vi "Launch Instruments.vi"(8 "error in (no error)":errorcluster, 11 "gController in":refnum<class "gController.lvclass">) -> (0 "error out":errorcluster, 3 "gController out":refnum<class "gController.lvclass">)   [LabVIEW 2017, in "Controller.lvlib" / "gController.lvclass"]
uses:
  gController.lvclass
  C:/Program Files (x86)/National Instruments/LabVIEW 2017/vi.lib/MSR Consulting, LLC/General Reuse/SuperActor/SuperActor.lvclass
  PAS/nPAS.lvclass
  C:/Program Files (x86)/National Instruments/LabVIEW 2017/vi.lib/MSR Consulting, LLC/General Reuse/Instrument/Instrument.lvclass
  <vilib>/MSR Consulting, LLC/General Reuse/PAS/Data/Main/PAS Data.lvclass
  C:/Program Files (x86)/National Instruments/LabVIEW 2017/vi.lib/MSR Consulting, LLC/General Reuse/Data/Data.lvclass
  CRD/gCRD.lvclass
  <vilib>/MSR Consulting, LLC/General Reuse/CRDS/Data/Main/CRDS Data.lvclass
  <vilib>/MSR Consulting, LLC/General Reuse/Instrument/Instrument.lvclass/Instrument.ctl
  <vilib>/MSR Consulting, LLC/General Reuse/Instrument/Actor/Instrument Actor.lvclass
  C:/Program Files (x86)/National Instruments/LabVIEW 2017/vi.lib/ActorFramework/Actor/Actor.lvclass
  Messages/Update Controller Data MSG/Update gController Data MSG.lvclass
  C:/Program Files (x86)/National Instruments/LabVIEW 2017/vi.lib/MSR Consulting, LLC/General Reuse/Generic Update Data MSG/Generic Update Data MSG.lvclass
  <vilib>/MSR Consulting, LLC/General Reuse/SuperActor/SuperActor.lvclass/SuperActor.ctl
  <vilib>/MSR Consulting, LLC/General Reuse/Instrument/Actor/Instrument Actor.lvclass/Instrument Actor.ctl
  <vilib>/MSR Consulting, LLC/General Reuse/SuperActor/Write ID.vi
  <vilib>/MSR Consulting, LLC/General Reuse/Instrument/Actor/Write Instr.vi
  <vilib>/MSR Consulting, LLC/General Reuse/Instrument/Actor/Write Update Data.vi
  <vilib>/MSR Consulting, LLC/General Reuse/Instrument/Write Data.vi
  <vilib>/MSR Consulting, LLC/General Reuse/SuperActor/SuperActor.lvclass
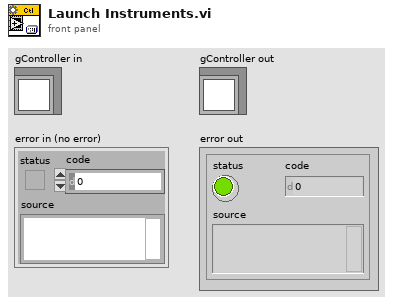
[diagram p1: front panel]
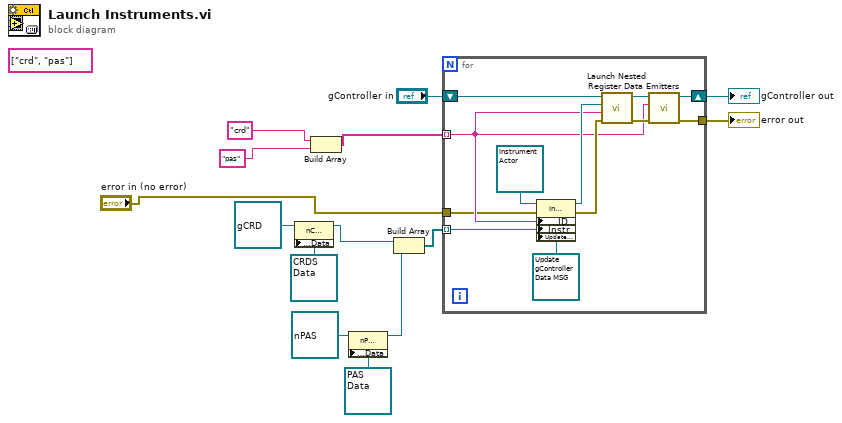
[diagram p0: block diagram]
diagram:
  (unwired) string[] ["crd", "pas"]
  n1 = property class="nCRD"(reference=refnum<class "gCRD.lvclass"> refnum ("gCRDS.lvlib:nCRD"), "Accessors:Data"=refnum<class "CRDS Data.lvclass"> refnum ("CRDS Lib.lvlib:CRDS")) -> (reference out=w4:refnum<class "gCRD.lvclass">)  [unwired: 1 in, 1 out]
  n2 = Build Array("crd" ("ID"), "pas" ("ID")) -> (w8:string[])
  n3 = property class="nPAS"(reference=refnum<class "nPAS.lvclass"> refnum ("gPAS Library.lvlib:nPAS"), "Accessors:Data"=refnum<class "PAS Data.lvclass"> refnum ("PAS Library.lvlib:PAS Data")) -> (reference out=w1:refnum<class "nPAS.lvclass">)  [unwired: 1 in, 1 out]
  n4 = Build Array(w4, w1) -> (w11:refnum<class "Instrument.lvclass">[])
  n5 = for {
    tunnel: [w18] -> w14
    shift-right: [w19] -> w13
    shift-left: "gController in" -> [w24]
    tunnel: w11 -> [w17] mode=indexing
    tunnel: w8 -> [w16] mode=indexing
    tunnel: "error in (no error)" -> [w15]
    n6 = property class="Instrument Actor"(reference=refnum<class "Instrument Actor.lvclass"> refnum ("Instrument Actor"), error in=w15, "Accessors:ID"=w16, "Instr"=w17, "Update Data"=refnum<class "Update gController Data MSG.lvclass"> refnum ("Controller.lvlib:Update gController Data MSG.lvclass")) -> (reference out=w25:refnum<class "Instrument Actor.lvclass">, error out=w23:errorcluster)
    n7 = call <vilib>:"Launch Nested.vi"("error in"=w23, "ID"=w16, "Nested Actor"=w25, "SuperActor in"=w24) -> ("error out"=w21:errorcluster, "SuperActor out"=w20:refnum<class "gController.lvclass">)  [unwired: 5 in, 1 out]
    n8 = call "Register Data Emitters.vi"("error in"=w21, "Emitter"=w16, "gController in"=w20) -> ("error out"=w18:errorcluster, "gController out"=w19:refnum<class "gController.lvclass">)  [unwired: 7 in]
  }
  "error out" <- w14
  "gController out" <- w13
